vi "Unpair Nodes.vi"(8 "error in (no error)":errorcluster, 10 "Node UID to Unpair":string, 11 "E2E editor node in":refnum<data-value>) -> (0 "error out":errorcluster, 3 "E2E editor node out":refnum<data-value>)   [LabVIEW 2015, in "E2E Tag Exchange editor node.lvclass"]
uses:
  E2E Tag Exchange editor node.lvclass
  Node LUT/Command.ctl
  Node LUT/Node LUT.lvlib
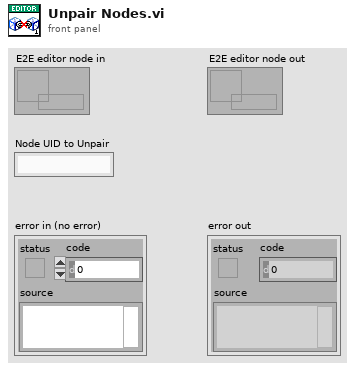
[diagram p1: front panel]
types:
  T1 = typedef "Node LUT.lvlib/Command.ctl" = enum16{"Initialize", "Add Node", "Remove Node", "Node Ref from UID", "List Nodes"}
  T2 = typedef "NISE_CEF_Node.lvclass/NodeRef.ctl" = refnum<data-value>
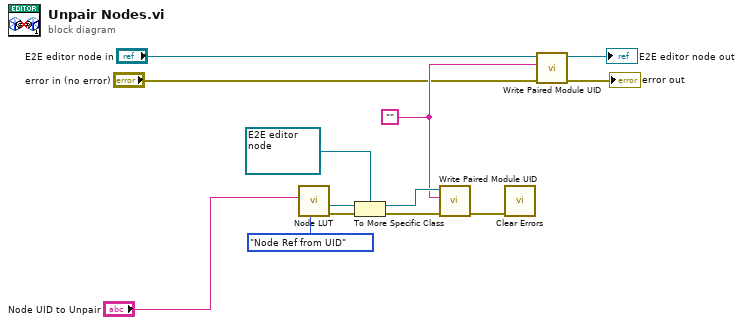
[diagram p0: block diagram]
diagram:
  w4 = ""
  n1 = call "Node LUT.vi"("Command"=Command."Node Ref from UID", "UID"="Node UID to Unpair") -> ("error out"=w11:errorcluster, "node ref"=w12:T2)  [unwired: 6 in, 2 out]
  n2 = To More Specific Class(target class=refnum<data-value> refnum, reference=w12, error in=w11) -> (specific class reference=w5:refnum<data-value>, error out=w3:errorcluster)
  n3 = call "Write Paired Module UID.vi"("error in (no error)"=w3, "Paired Module UID"=w4, "E2E editor node in"=w5) -> ("error out"=w1:errorcluster)  [unwired: 7 in, 1 out]
  n4 = call <vilib>:"Clear Errors.vi"("error in (no error)"=w1) -> ()  [unwired: 5 in, 2 out]
  n5 = call "Write Paired Module UID.vi"("error in (no error)"="error in (no error)", "Paired Module UID"=w4, "E2E editor node in"="E2E editor node in") -> ("error out"=→"error out":errorcluster, "E2E editor node out"=→"E2E editor node out":refnum<data-value>)  [unwired: 7 in]
